vi "CR-SaveImageCCD4暂存.vi"(6 "类型":string(combo)="Front conveyor", 8 "error in (no error)":errorcluster, 9 "Image in":T1(plugin-control), 10 "布尔":bool=TRUE, 11 "基路径":path) -> (0 "error out":errorcluster)   [LabVIEW 2017]
panel:
  in  "CCD Name":string(combo)="CCD4"
  out "连接的字符串":string
  # "D:\\Data\\History Image\\20190228\\CCD3\\Image"
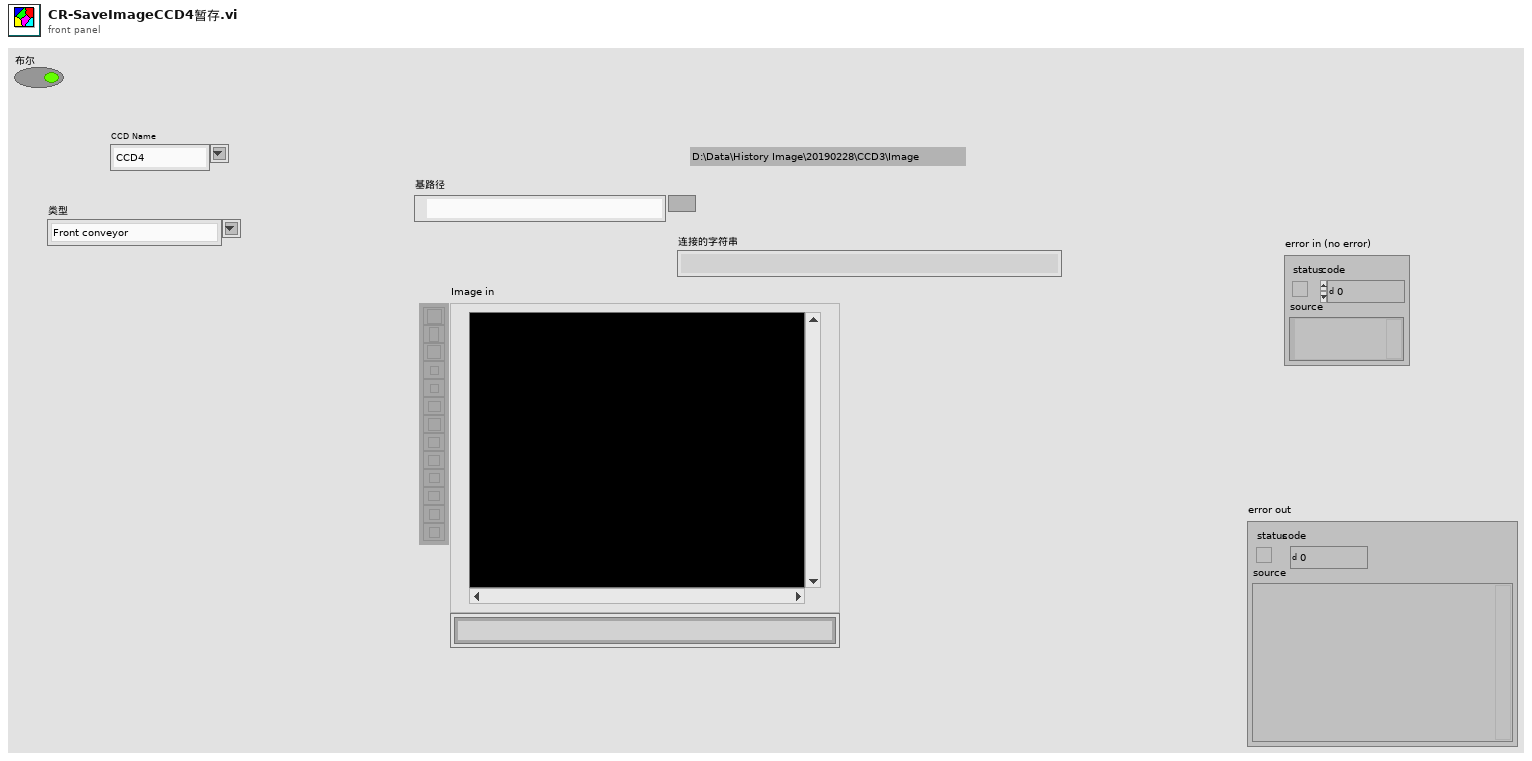
[diagram p1: front panel]
types:
  T1 = typedef "IMAQ Image.ctl" = refnum<image>
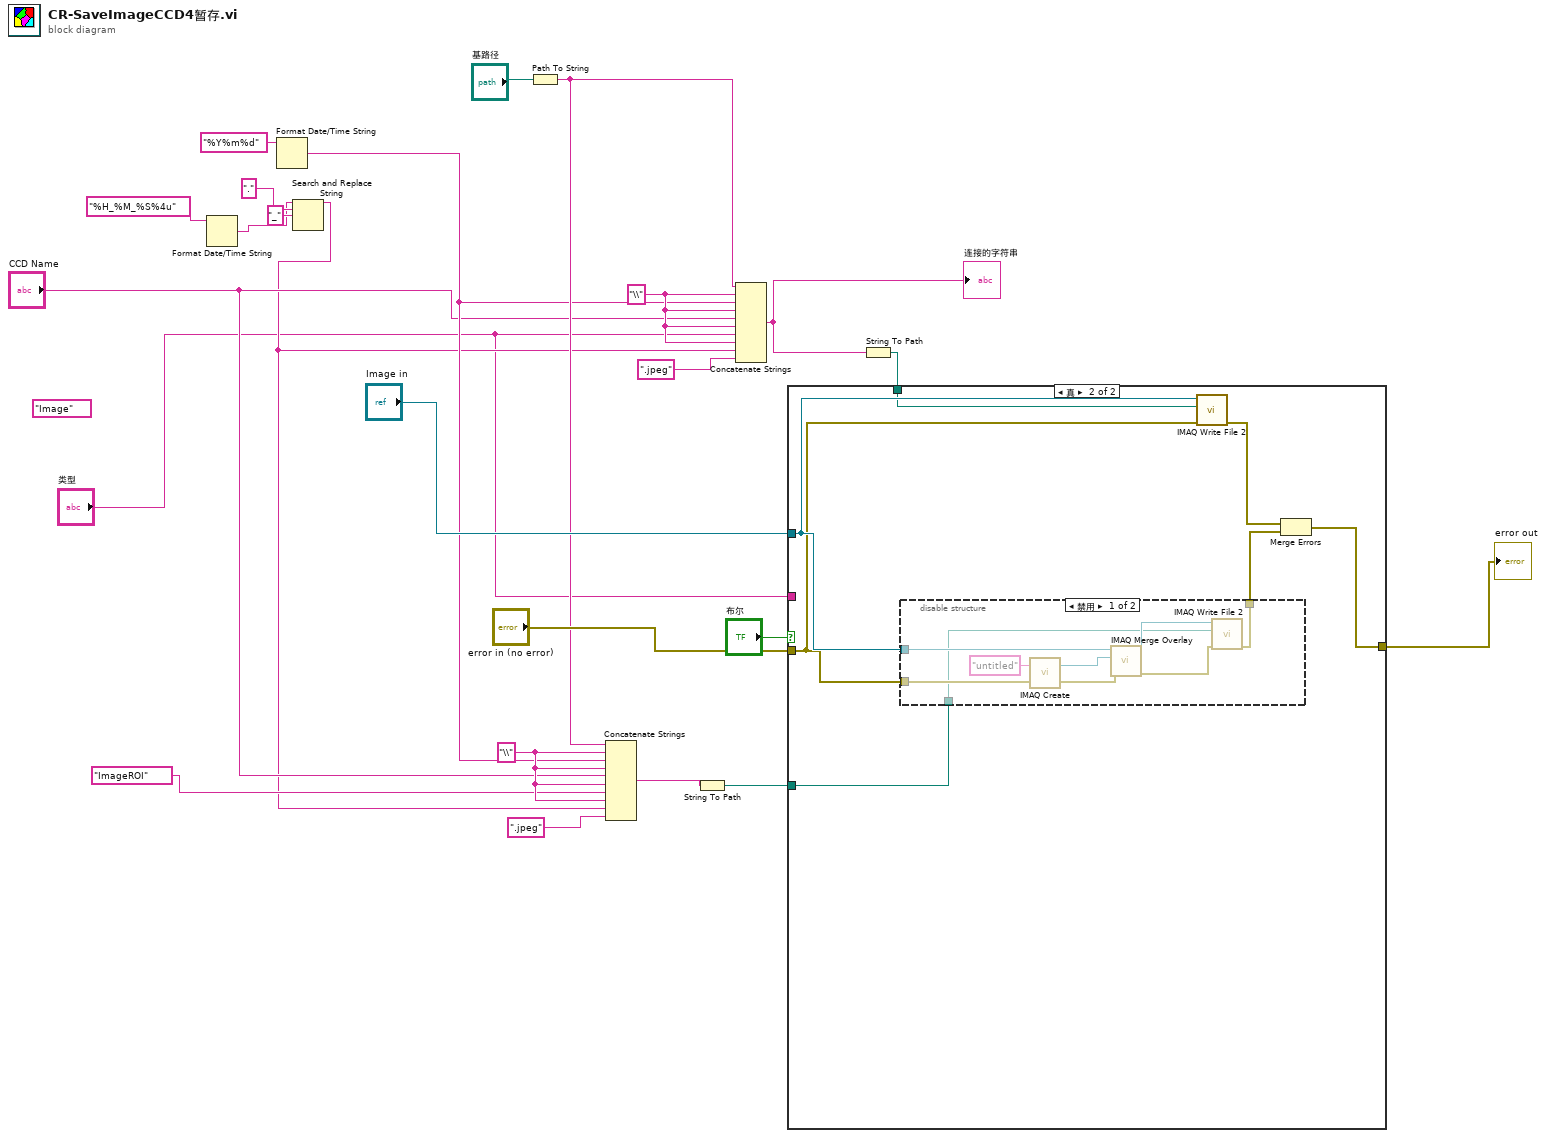
[diagram p0: block diagram]
diagram:
  (unwired) "Image" ("类型")
  w13 = "\\" ("字符串")
  w16 = "\\" ("字符串")
  n1 = Format Date/Time String(time format string (%c)="%H_%M_%S%4u" ("时间格式字符串(%c)")) -> (date/time string=w3:string)  [unwired: 2 in]
  n2 = Format Date/Time String(time format string (%c)="%Y%m%d" ("时间格式字符串(%c)")) -> (date/time string=w10:string)  [unwired: 2 in]
  n3 = Search and Replace String(input string=w3, search string="." ("搜索字符串"), replace string="_" ("替换字符串(\"\")")) -> (result string=w2:string)  [unwired: 5 in, 3 out]
  n4 = Path To String(path="基路径") -> (string=w11:string)
  n5 = Concatenate Strings(w11, w13, w10, w13, "CCD Name", w13, "ImageROI" ("类型"), w13, w2, ".jpeg" ("字符串")) -> (w7:string)
  n6 = String To Path(string=w7) -> (path=w6:path)
  n7 = Concatenate Strings(w11, w16, w10, w16, "CCD Name", w16, "类型", w16, w2, ".jpeg" ("字符串")) -> (w22:string)
  "连接的字符串" <- w22
  n8 = String To Path(string=w22) -> (path=w18:path)
  n9 = case shown="真" "布尔" {
    tunnel: "Image in" -> [_ w32]
    tunnel: "error in (no error)" -> [w25 w31]
    tunnel: w18 -> [_ w26]
    tunnel: [w25 w28] -> w15
    tunnel: "类型" -> [_ _]
    tunnel: w6 -> [_ w27]
    frame False {
    }
    frame True {
      n10 = disable-structure shown="禁用" {
        disable-tunnel: w32 -> [w41 _]
        disable-tunnel: w31 -> [w40 _]
        disable-tunnel: [w34 _] -> w30
        disable-tunnel: w27 -> [w33 _]
        frame Disabled {
          n11 = call "IMAQ Create"("Image Name"="untitled", "error in (no error)"=w40) -> ("New Image"=w36:T1, "error out"=w35:errorcluster)  [unwired: 3 in]
          n12 = call "IMAQ Merge Overlay"("error in (no error)"=w35, "Image Dst"=w36, "Image Src"=w41) -> ("error out"=w38:errorcluster, "Image Dst Out"=w39:T1)  [unwired: 7 in]
          n13 = call-poly "IMAQ Write File 2"("error in (no error)"=w38, "File Path"=w33, "Image"=w39) -> ("error out"=w34:errorcluster)  [unwired: 7 in, 1 out]
        }
        frame Enabled {
        }
      }
      n14 = call-poly "IMAQ Write File 2"("error in (no error)"=w31, "File Path"=w26, "Image"=w32) -> ("error out"=w29:errorcluster)  [unwired: 7 in, 1 out]
      n15 = Merge Errors(w29, w30) -> (w28:errorcluster)
    }
  }
  "error out" <- w15
